vi "ReplaceIllegalCharacters.vi"(11 "input string":string) -> (3 "result string":string)   [LabVIEW 2017, in "Tdms.lvlib"]
uses:
  <vilib>/addons/InsightCM/Utilities/Tdms/Tdms.lvlib
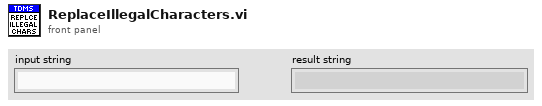
[diagram p1: front panel]
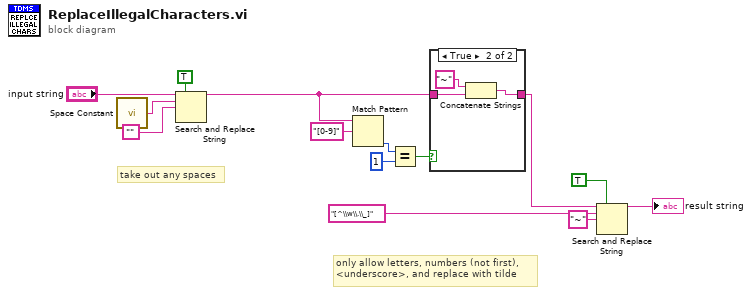
[diagram p0: block diagram]
diagram:
  # "take out any spaces"
  # "only allow letters, numbers (not first), \n<underscore>, and replace with tilde"
  n1 = call <vilib>:"Space Constant.vi"() -> ("String"=w2:string)
  n2 = Search and Replace String(replace all?=TRUE ("replace all? (F)"), input string="input string", search string=w2, replace string="") -> (result string=w3:string)  [unwired: 4 in, 3 out]
  n3 = Match Pattern(string=w3, regular expression="[0-9]") -> (offset past match=w8:i32)  [unwired: 1 in, 3 out]
  n4 = Equal?(x=w8, y=1) -> (x = y?=w6:bool)
  n5 = case shown="True" w6 {
    tunnel: w3 -> [w15 w18]
    tunnel: [w15 w16] -> w10
    frame False {
    }
    frame True {
      n6 = Concatenate Strings("~" ("replace string (\"\")"), w18) -> (w16:string)
    }
  }
  n7 = Search and Replace String(replace all?=TRUE ("replace all? (F)"), input string=w10, search string="[^\\w\\.\\_]" ("regular expression"), replace string="~" ("replace string (\"\")")) -> (result string=→"result string":string)  [unwired: 4 in, 3 out]
